vi "Next Value - NT Scalar.vi"(8 "error in (no error)":errorcluster, 9 "timeout":dbl[unit]=1.0, 10 "default value":refnum<class "NT Scalar.lvclass">, 11 "Subscription in":refnum<class "Subscription.lvclass">) -> (0 "error out":errorcluster, 1 "timed out?":bool, 2 "value":refnum<class "NT Scalar.lvclass">, 3 "Subscription out":refnum<class "Subscription.lvclass">, 5 "PV name":string)   [LabVIEW 2020, in "PV Access.lvlib" / "PVA Client.lvlib" / "Subscription.lvclass"]
uses:
  Subscription.lvclass
  PV Data/NT Scalar/NT Scalar.lvclass
  C:/Users/eyw68381/source/repos/pvaccess-labview/labview/source/PV Data/Base/Base.lvclass
  Subscription.lvclass/Subscription.ctl
  PV Data/PV Data/PV Data.lvclass
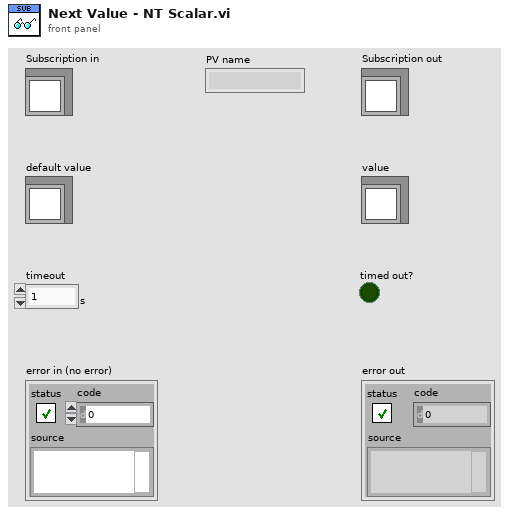
[diagram p1: front panel]
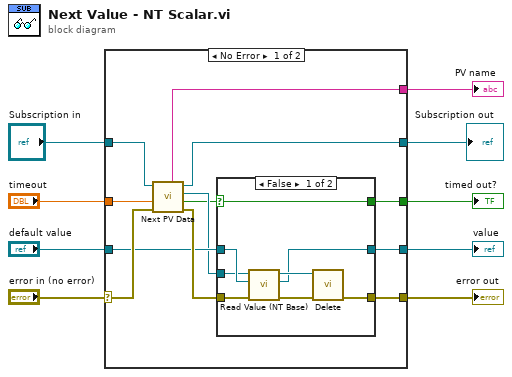
[diagram p0: block diagram]
diagram:
  n1 = case shown="No Error" "error in (no error)" {
    selector: "error in (no error)" -> [w19 w35]
    tunnel: [w12 w35] -> w8
    tunnel: [w20 w34] -> w6
    tunnel: "Subscription in" -> [w21 w34]
    tunnel: "timeout" -> [w18 _]
    tunnel: "default value" -> [w15 w33]
    tunnel: [w13 w33] -> w1
    tunnel: [w10 _] -> w3
    tunnel: [w17 _] -> w2
    frame No Error {
      n2 = call "Next PV Data.vi"("error in (no error)"=w19, "timeout"=w18, "Subscription in"=w21) -> ("error out"=w16:errorcluster, "timed out?"=w11:bool, "PV Data"=w14:refnum<class "PV Data.lvclass">, "Subscription out"=w20:refnum<class "Subscription.lvclass">, "PV name"=w17:string)  [unwired: 4 in]
      n3 = case shown="False" w11 {
        selector: w11 -> [w22 w32]
        tunnel: w16 -> [w29 w30]
        tunnel: w15 -> [w26 w31]
        tunnel: w14 -> [w25 _]
        tunnel: [w24 w31] -> w13
        tunnel: [w23 w30] -> w12
        tunnel: [w22 w32] -> w10
        frame False {
          n4 = call "Read Value (NT Base).vi"("error in (no error)"=w29, "default value"=w26, "PV Data in"=w25) -> ("error out"=w28:errorcluster, "value"=w24:refnum<class "NT Scalar.lvclass">, "PV Data out"=w27:refnum<class "PV Data.lvclass">)  [unwired: 6 in]
          n5 = call "Delete.vi"("error in (no error)"=w28, "PV Data in"=w27) -> ("error out"=w23:errorcluster)  [unwired: 9 in]
        }
        frame True {
        }
      }
    }
    frame Error {
    }
  }
  "error out" <- w8
  "Subscription out" <- w6
  "value" <- w1
  "timed out?" <- w3
  "PV name" <- w2
